vi "Write AI Configuration.vi"(8 "error in (no error)":errorcluster, 10 "AI Configuration":T1 {"input terminal configuration" items=["default"=-1, "RSE"=10083, "NRSE"=10078, "Differential"=10106, "Pseudodifferential"=12529]; "AI.Coupling" items=["AC"=10045, "DC"=10050, "GND"=10066]}, 11 "Lockin.DAQ":refnum<class "Lockin.DAQ.lvclass">) -> (0 "error out":errorcluster, 3 "Lockin.DAQ out":refnum<class "Lockin.DAQ.lvclass">)   [LabVIEW 2016, in "Lockin.DAQ.lvclass"]
uses:
  Lockin.DAQ.lvclass
  Typedefs/AI.config-array.ctl
  Typedefs/AI.config-cluster.ctl
  Typedefs/AI.coupling-enum.ctl
  Typedefs/446xAI-enum.ctl
  Typedefs/DAQType-enum.ctl
  Lockin.DAQ.lvclass/Lockin.DAQ.ctl
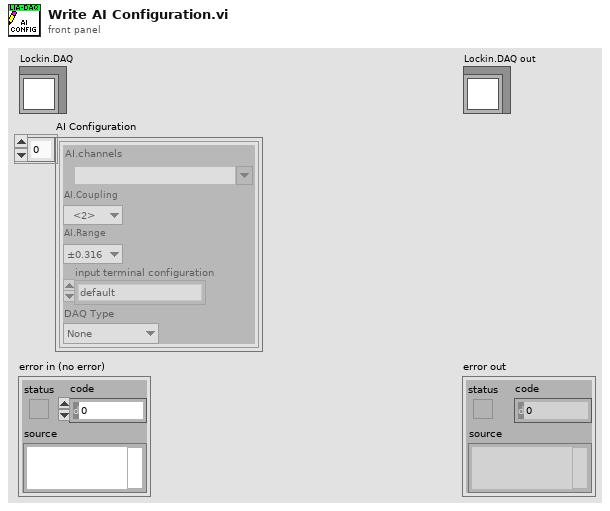
[diagram p1: front panel]
types:
  T1 = typedef "Lockin.DAQ.lvclass/AI.config-array.ctl" = T2[]
  T2 = typedef "Lockin.DAQ.lvclass/AI.config-cluster.ctl" = cluster{"AI.channels":tag, "AI.Coupling":T3, "AI.Range":T4, "input terminal configuration":i32, "DAQ Type":T5}
  T3 = typedef "Lockin.DAQ.lvclass/AI.coupling-enum.ctl" = u16
  T4 = typedef "Lockin.DAQ.lvclass/446xAI-enum.ctl" = enum16{"±0.316", "±1.00", "±3.16", "±10.0", "±31.6", "±42.4"}
  T5 = typedef "Lockin.DAQ.lvclass/DAQType-enum.ctl" = enum16{"None", "USB 4431", "PXI 446x"}
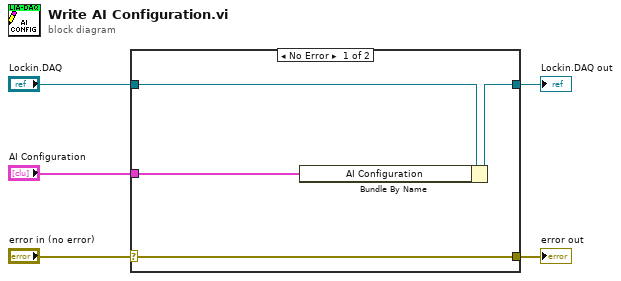
[diagram p0: block diagram]
diagram:
  n1 = case shown="No Error" "error in (no error)" {
    selector: "error in (no error)" -> [w9 w10]
    tunnel: [w9 w10] -> w4
    tunnel: [w7 w11] -> w2
    tunnel: "Lockin.DAQ" -> [w8 w11]
    tunnel: "AI Configuration" -> [w6 _]
    frame No Error {
      n2 = Bundle By Name(cluster=w8, "AI Configuration"=w6) -> (w7:refnum<class "Lockin.DAQ.lvclass">)
    }
    frame Error {
    }
  }
  "error out" <- w4
  "Lockin.DAQ out" <- w2
